vi "Error Message.vi"() -> (0 "logical AND":bool, 2 "Error":string)   [LabVIEW 2015]
uses:
  Galobal variable_TI.vi
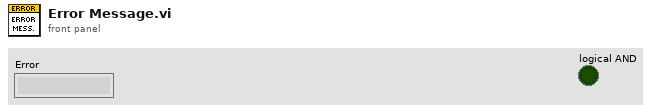
[diagram p1: front panel]
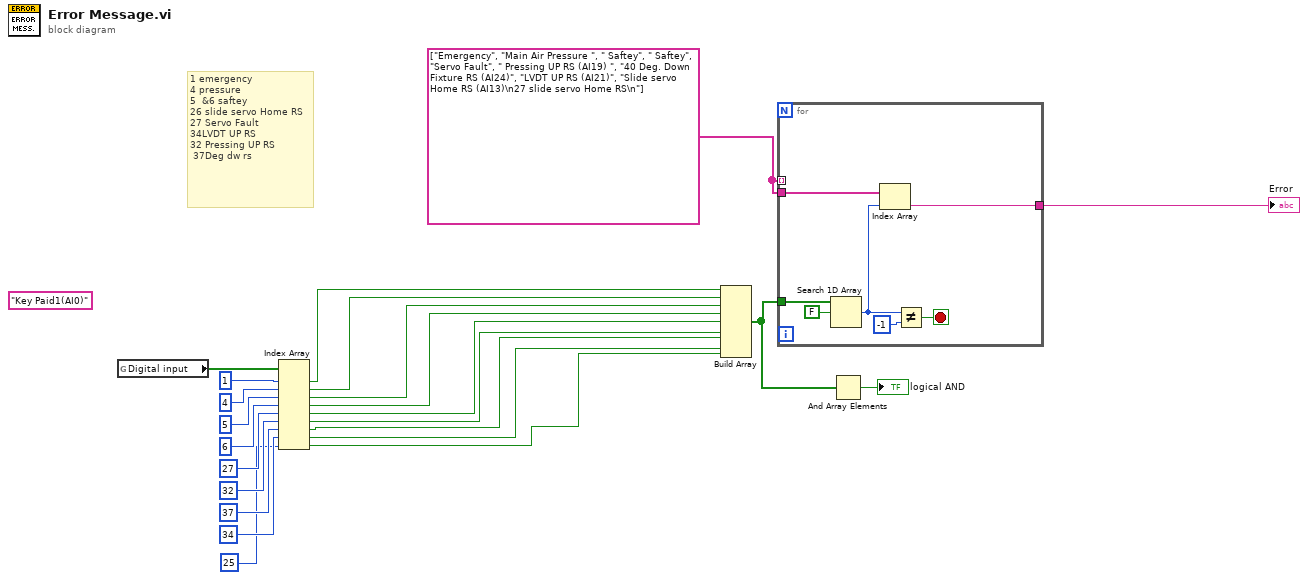
[diagram p0: block diagram]
diagram:
  (unwired) "Key Paid1(AI0)"
  w23 = string[] ["Emergency", "Main Air Pressure ", " Saftey", " Saftey", "Servo Fault", " Pressing UP RS (AI19) ", "40 Deg. Down Fixture RS (AI24)", "LVDT UP RS (AI21)", "Slide servo Home RS (AI13)\n27 slide servo Home RS\n"]
  # "1 emergency\n4 pressure\n5  &6 saftey\n26 slide servo Home RS\n27 Servo Fault\n34LVDT UP RS\n32 Pressing UP RS \n 37Deg dw rs"
  n1 = global read "Galobal variable_TI.vi" "Digital input"() -> (w19:bool[])
  n2 = Index Array(array=w19, index #1=1 ("index"), index #2=4 ("index"), index #3=5 ("index"), index #4=6 ("index"), index #5=27 ("index"), index #6=32 ("index"), index #7=37 ("index"), index #8=34 ("index"), index #9=25 ("index")) -> (element #1=w21:bool, element #2=w11:bool, element #3=w10:bool, element #4=w9:bool, element #5=w3:bool, element #6=w8:bool, element #7=w7:bool, element #8=w6:bool, element #9=w4:bool)
  n3 = Build Array(w21, w11, w10, w9, w3, w8, w7, w6, w4) -> (w2:bool[])
  n4 = for {
    tunnel: w23 -> [_] mode=indexing
    tunnel: w23 -> [w27]
    tunnel: w2 -> [w29]
    tunnel: [w25] -> w22
    stop <- w28 stop-if-true
    n5 = Search 1D Array(1D array=w29, element=FALSE) -> (index of element=w26:i32)  [unwired: 1 in]
    n6 = Index Array(array=w27, index=w26) -> (element=w25:string)
    n7 = Not Equal?(x=w26, y=-1) -> (x != y?=w28:bool)
  }
  "Error" <- w22
  n8 = And Array Elements(Boolean array=w2) -> (logical AND=→"logical AND":bool)
